vi "ex_PPGetValue.vi"(0 "Control Data":T1, 11 "Control:":string="Simulated Analog Input") -> (4 "Value":variant, 15 "Found":bool)   [LabVIEW 2017]
doc: "Specifies whether a particular control is found on both the Express VI and its value on the property page given references to both VIs and their controls, the Control Data array, and the name of the control you are looking for."
uses:
  <vilib>/express/express shared/propPageData.ctl
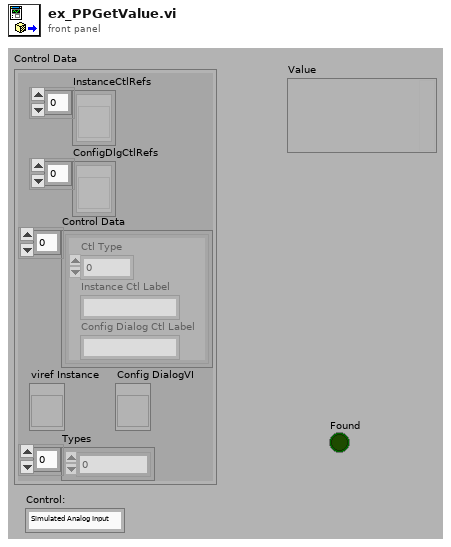
[diagram p1: front panel]
types:
  T1 = typedef "propPageData.ctl" = cluster{"InstanceCtlRefs":refnum<vi>[], "ConfigDlgCtlRefs":refnum<vi>[], "Control Data":cluster{"Ctl Type":u16, "Instance Ctl Label":string, "Config Dialog Ctl Label":string}[], "viref Instance":refnum<vi>, "Types":i32[], "Config DialogVI":refnum<vi>}
  T2 = cluster{"Ctl Type":u16, "Instance Ctl Label":string, "Config Dialog Ctl Label":string}[]
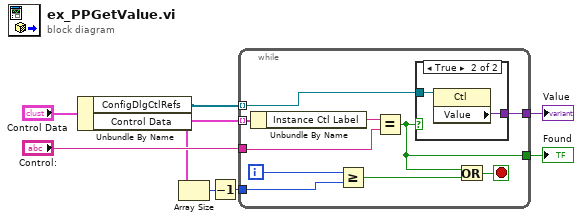
[diagram p0: block diagram]
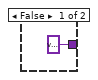
[diagram p2: hidden frame]
diagram:
  n1 = Unbundle By Name("Control Data") -> ("ConfigDlgCtlRefs"=w7:refnum<vi>[], "Control Data"=w4:T2)
  n2 = Array Size(array=w4) -> (size(s)=w3:i32)
  n3 = Decrement(x=w3) -> (x-1=w2:i32)
  n4 = while {
    tunnel: w4 -> [w18] mode=indexing
    tunnel: w7 -> [w17] mode=indexing
    tunnel: "Control:" -> [w16]
    tunnel: [w15] -> w5
    tunnel: w2 -> [w10]
    tunnel: [w12] -> w1
    i -> [w9]
    stop <- w13 stop-if-true
    n5 = Unbundle By Name(w18) -> ("Instance Ctl Label"=w14:string)
    n6 = Greater Or Equal?(x=w9, y=w10) -> (x >= y?=w11:bool)
    n7 = Equal?(x=w14, y=w16) -> (x = y?=w12:bool)
    n8 = case shown="True" w12 {
      tunnel: w17 -> [_ w21]
      tunnel: [variant ("Value") w20] -> w15
      frame False {
      }
      frame True {
        n9 = property class="Ctl"(reference=w21) -> ("Value"=w20:variant)  [unwired: 1 in, 2 out]
      }
    }
    n10 = Or(x=w12, y=w11) -> (x .or. y?=w13:bool)
  }
  "Value" <- w5
  "Found" <- w1
